vi "选择打印文件.vi"() -> ()   [LabVIEW 2014]
panel:
  in  "选择打印文件":path
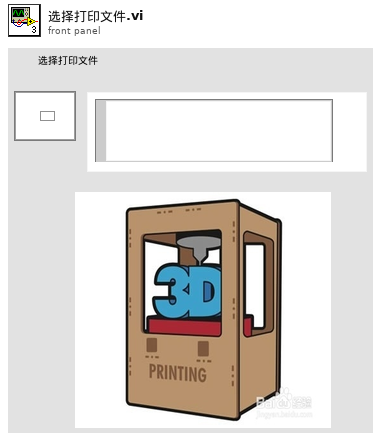
[diagram p1: front panel]
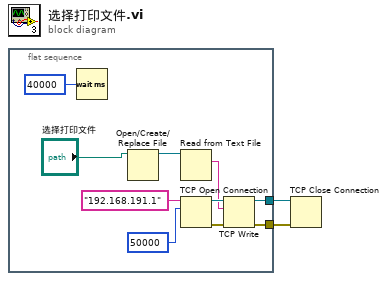
[diagram p0: block diagram]
diagram:
  n1 = flat-sequence {
    tunnel: [w10] -> w2
    tunnel: [w5] -> w1
    frame #0 {
      n2 = Wait (ms)(milliseconds to wait=u32 40000) -> ()  [unwired: 1 out]
      n3 = Open/Create/Replace File(file path (use dialog)="选择打印文件") -> (refnum out=w11:refnum<file>)  [unwired: 5 in, 2 out]
      n4 = Read from Text File(file (use dialog)=w11) -> (text=w6:string)  [unwired: 3 in, 3 out]
      n5 = TCP Open Connection(address="192.168.191.1", remote port or service name=u16 50000) -> (connection ID=w12:refnum<k5>, error out=w9:errorcluster)  [unwired: 3 in]
      n6 = TCP Write(connection ID=w12, data in=w6, error in (no error)=w9) -> (connection ID out=w10:refnum<k5>, error out=w5:errorcluster)  [unwired: 1 in, 1 out]
    }
  }
  n7 = TCP Close Connection(connection ID=w2, error in (no error)=w1) -> ()  [unwired: 1 in, 2 out]
